vi "Get Setting.vi"(8 "error in (no error)":errorcluster, 9 "Device and Axis":string, 10 "Setting":string, 11 "VISA resource name":refnum<visa-resource-name>) -> (0 "error out":errorcluster, 1 "Response Bundle Array":T1(array[cluster]), 2 "Response String Array":string[](array[string]), 3 "VISA resource name out":refnum<visa-resource-name>, 4 "First Response Data":string, 5 "Number of Replies":i32)   [LabVIEW 2021, in "Zaber A Series.lvlib"]
doc: "Reads a setting from the device. Omitting the Device and Axis will return the settings of all connected devices. See a list of settings available here: http://www.zaber.com/wiki/Manuals/ASCII_Protocol_Manual#Device_Settings. You do not need to include the 'get' command with this VI, you only need to input the setting you would like to check. \n\nThe Detect Devices VI is designed to provide an easy list of valid Device and Axis inputs. \n\nAn array containing the complete strings of the responses is returned on the Response String Array output, and the details of the format of the response are described here: http://www.zaber.com/wiki/Manuals/ASCII_Protocol_Manual#Replies. This VI also parses the strings, bundles the components, and returns them as an array of bundles on the Response Bundle Array pin. Additionally a pin returns the number of responses received. \n\nThis VI requires that the Initialize VI has been called with the same serial port."
uses:
  Zaber A Series.lvlib
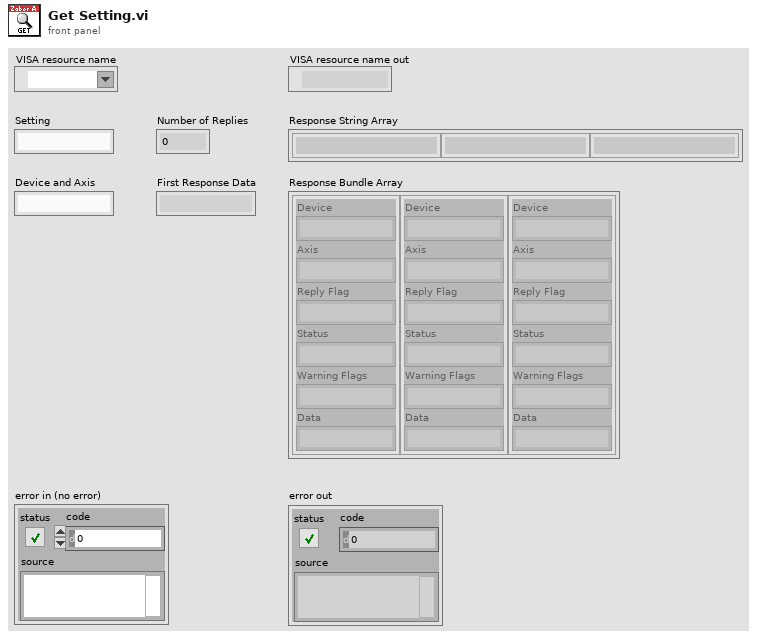
[diagram p1: front panel]
types:
  T1 = cluster{"Device":string, "Axis":string, "Reply Flag":string, "Status":string, "Warning Flags":string, "Data":string}[]
  T2 = cluster{"Device":string, "Axis":string, "Reply Flag":string, "Status":string, "Warning Flags":string, "Data":string}
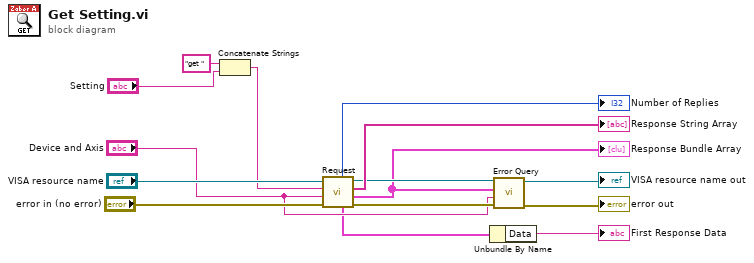
[diagram p0: block diagram]
diagram:
  n1 = Concatenate Strings("get " ("string"), "Setting") -> (w12:string)
  n2 = call "Request.vi"("error in (no error)"="error in (no error)", "Device and Axis"="Device and Axis", "Command String"=w12, "VISA resource name"="VISA resource name") -> ("error out"=w7:errorcluster, "Response Bundle Array"=w4:T1, "Response String Array"=→"Response String Array":string[], "VISA resource name out"=w8:refnum<visa-resource-name>, "First Response Bundle"=w2:T2, "Number of Replies"=→"Number of Replies":i32)  [unwired: 2 in]
  "Response Bundle Array" <- w4
  n3 = Unbundle By Name(w2) -> ("Data"=→"First Response Data":string)
  n4 = call "Error Query.vi"("error in (no error)"=w7, "Device and Axis"="Device and Axis", "Previous Response Bundle Array"=w4, "VISA resource name"=w8) -> ("error out"=→"error out":errorcluster, "VISA resource name out"=→"VISA resource name out":refnum<visa-resource-name>)  [unwired: 4 in, 2 out]
